vi "FFGETone.vi"(3 "pixel":u32=600, 5 "lfkt":i32=1) -> (0 "esc":bool, 1 "space":bool, 2 "Data Values":u16[](graph))   [LabVIEW 2014]
uses:
  ESLSCDLL.dll
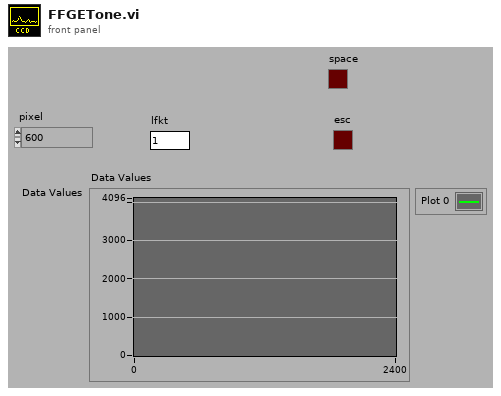
[diagram p1: front panel]
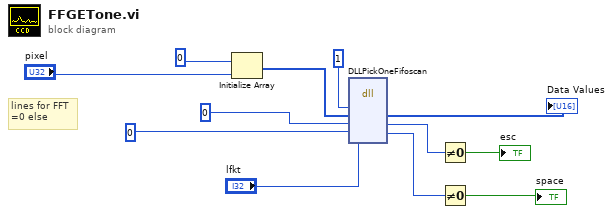
[diagram p0: block diagram]
diagram:
  # "lines for FFT\n=0 else"
  n1 = Initialize Array(u16 0, "pixel") -> (w10:u16[])
  n2 = dll-call lib="C:/Users/Gerhard/Documents/New64/lv/1cam/board.vis/ESLSCDLL.dll" fn="DLLPickOneFifoscan"("drv"=u32 1, "pdioden"=w10, "abbr"=u8 0, "space"=u8 0, "fkt"="lfkt") -> ("pdioden"=→"Data Values":u16[], "abbr"=w4:u8, "space"=w3:u8)  [unwired: 6 in, 2 out]
  n3 = Not Equal To 0?(x=w4) -> (x != 0?=→"esc":bool)
  n4 = Not Equal To 0?(x=w3) -> (x != 0?=→"space":bool)
